vi "Release System.vi"(8 "error in (no error)":errorcluster, 11 "System Configuration":T1) -> (0 "error out":errorcluster)   [LabVIEW 2024]
doc: "Releases the server process in the shared variable engine."
uses:
  Controls/Server/System Configuration.ctl
  Controls/Server/Subsystem Configuration.ctl
  <vilib>/lvdsc/NI_DSC.lvlib
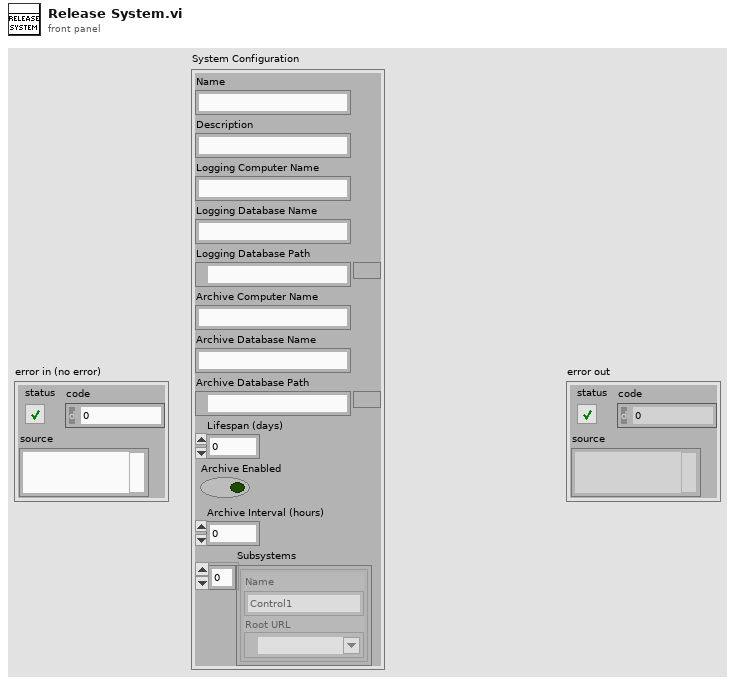
[diagram p1: front panel]
types:
  T1 = typedef "System Configuration.ctl" = cluster{"Name":string, "Description":string, "Logging Computer Name":string, "Logging Database Name":string, "Logging Database Path":path, "Archive Computer Name":string, "Archive Database Name":string, "Archive Database Path":path, "Lifespan (days)":u32, "Archive Enabled":bool, "Archive Interval (hours)":u32, "Subsystems":T2[]}
  T2 = typedef "Subsystem Configuration.ctl" = cluster{"Name":string, "Root URL":refnum<k21>}
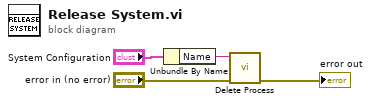
[diagram p0: block diagram]
diagram:
  n1 = Unbundle By Name("System Configuration") -> ("Name"=w3:string)
  n2 = call <vilib>:"Delete Process.vi"("error in (no error)"="error in (no error)", "process name"=w3) -> ("error out"=→"error out":errorcluster)  [unwired: 9 out]
